vi "Open Connection.vi"(8 "error in (no error)":errorcluster, 10 "DatabaseFilePath":string, 11 "sqlite in":refnum<class "sqlite3.lvclass">) -> (0 "error out":errorcluster, 3 "sqlite out":refnum<class "sqlite3.lvclass">)   [LabVIEW 2020, in "sqlite3.lvlib" / "sqlite3.lvclass"]
uses:
  sqlite3.lvclass
  sqlite3.lvclass/sqlite3.ctl
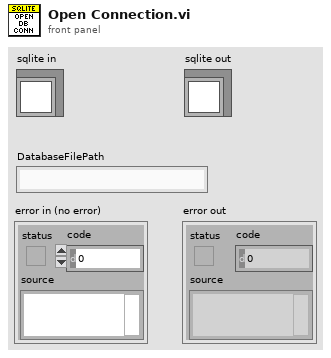
[diagram p1: front panel]
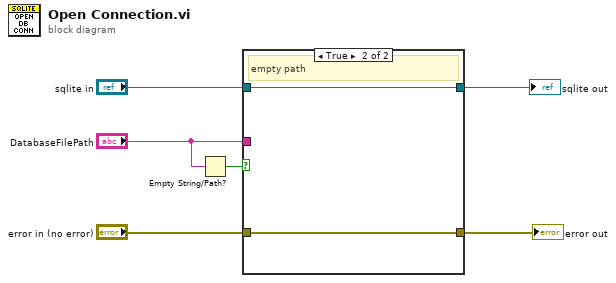
[diagram p0: block diagram]
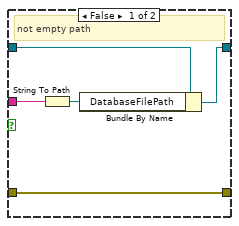
[diagram p2: hidden frame]
diagram:
  n1 = Empty String/Path?(string/path="DatabaseFilePath") -> (empty?=w3:bool)
  n2 = case shown="True" w3 {
    tunnel: "sqlite in" -> [w11 w13]
    tunnel: [w10 w13] -> w5
    tunnel: "DatabaseFilePath" -> [w9 _]
    tunnel: "error in (no error)" -> [w7 w12]
    tunnel: [w7 w12] -> w1
    frame False {
      # "not empty path"
      n3 = String To Path(string=w9) -> (path=w8:path)
      n4 = Bundle By Name(cluster=w11, "DatabaseFilePath"=w8) -> (w10:refnum<class "sqlite3.lvclass">)
    }
    frame True {
      # "empty path"
    }
  }
  "error out" <- w1
  "sqlite out" <- w5
